vi "Save start time.vi"(8 "error in (no error)":errorcluster, 10 "Start time":timestamp, 11 "file refs":T1 {"file" format="%.0x"}) -> (0 "error out":errorcluster, 3 "file refs out":T1 {"file" format="%.0x"})   [LabVIEW 2013]
uses:
  File refs.ctl
  <vilib>/addons/h5labview2/base/hid_t.ctl
  <vilib>/addons/h5labview2/base/lib_path.vi
  <vilib>/addons/h5labview2/base/H5Equery.vi
  <vilib>/addons/h5labview2/attrib/H5Awrite.llb/H5Awrite.xnode
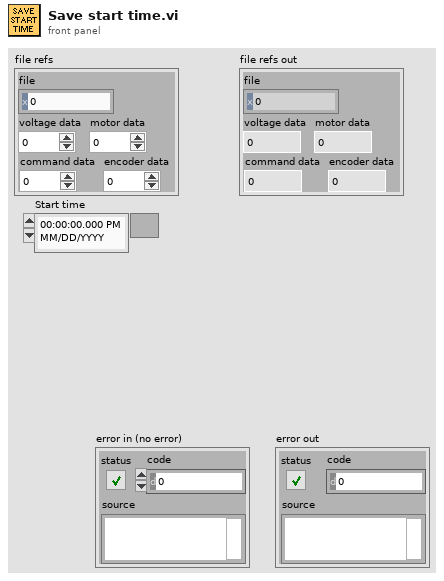
[diagram p1: front panel]
types:
  T1 = typedef "File refs.ctl" = cluster{"file":T2, "voltage data":i32, "motor data":i32, "command data":i32, "encoder data":i32}
  T2 = typedef "hid_t.ctl" = i32
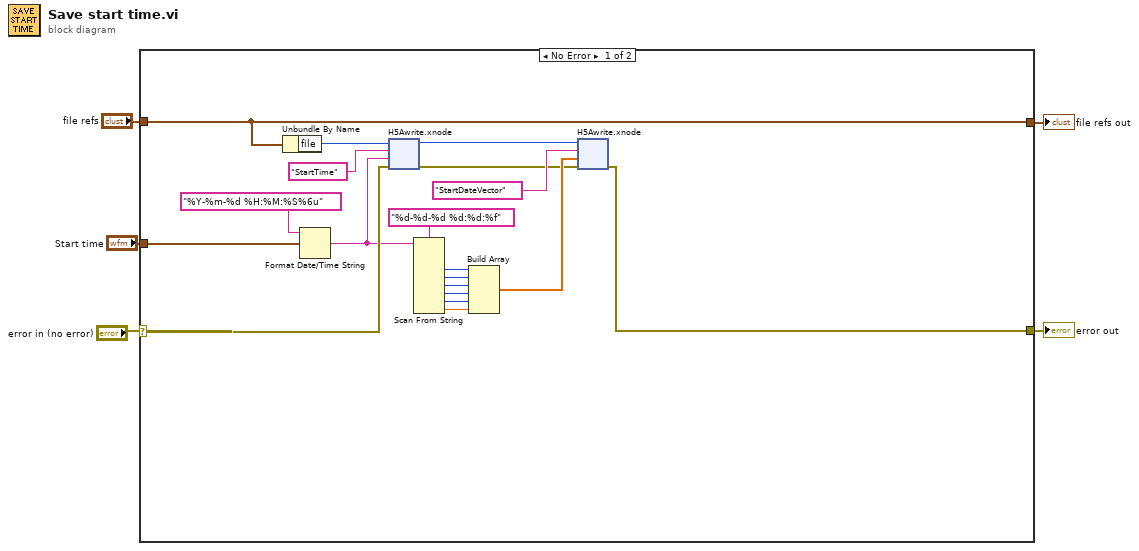
[diagram p0: block diagram]
diagram:
  n1 = case shown="No Error" "error in (no error)" {
    selector: "error in (no error)" -> [w19 w61]
    tunnel: "file refs" -> [w24 w62]
    tunnel: [w6 w61] -> w3
    tunnel: [w24 w62] -> w2
    tunnel: "Start time" -> [w21 _]
    frame No Error {
      n2 = Unbundle By Name(w24) -> ("file"=w23:T2)
      n3 = Format Date/Time String(time format string (%c)="%Y-%m-%d %H:%M:%S%6u", seconds (now)=w21) -> (date/time string=w18:string)  [unwired: 1 in]
      n4 = xnode "H5Awrite.xnode"("error in (no error)"=w19, "data"=w18, "attrib name"="StartTime", "ref in"=w23) -> ("error out"=w7:errorcluster, "ref out"=w10:T2)  [unwired: 3 in, 1 out]
      n5 = Scan From String(format string="%d-%d-%d %d:%d:%f", input string=w18) -> (output 1=w16:i32, output 2=w15:i32, output 3=w14:i32, output 4=w13:i32, output 5=w12:i32, output 6=w11:dbl)  [unwired: 8 in, 3 out]
      n6 = Build Array(w16, w15, w14, w13, w12, w11) -> (w8:dbl[])
      n7 = xnode "H5Awrite.xnode"("error in (no error)"=w7, "data"=w8, "attrib name"="StartDateVector", "ref in"=w10) -> ("error out"=w6:errorcluster)  [unwired: 3 in, 2 out]
    }
    frame Error {
    }
  }
  "error out" <- w3
  "file refs out" <- w2
